vi "HDI Pat Match Full with Move TR.vi"(5 "controller in":refnum<k24>, 11 "error in":errorcluster) -> (4 "In Range?":bool, 8 "x rel move":dbl, 10 "y rel move":dbl, 14 "Horizontal vector":dbl[](array[numeric]), 15 "error out":errorcluster)   [LabVIEW 2011]
uses:
  C:/Users/Admin/Desktop/Gantry Code Transfer/source/Code Transfer/Aerotech.A3200.dll
  Aerotech.A3200.dll
  <vilib>/vision/driver/NI_Vision_Acquisition_Software.lvlib
panel:
  out "Angle Between Lines":dbl
  out "Diagnostic Log":string
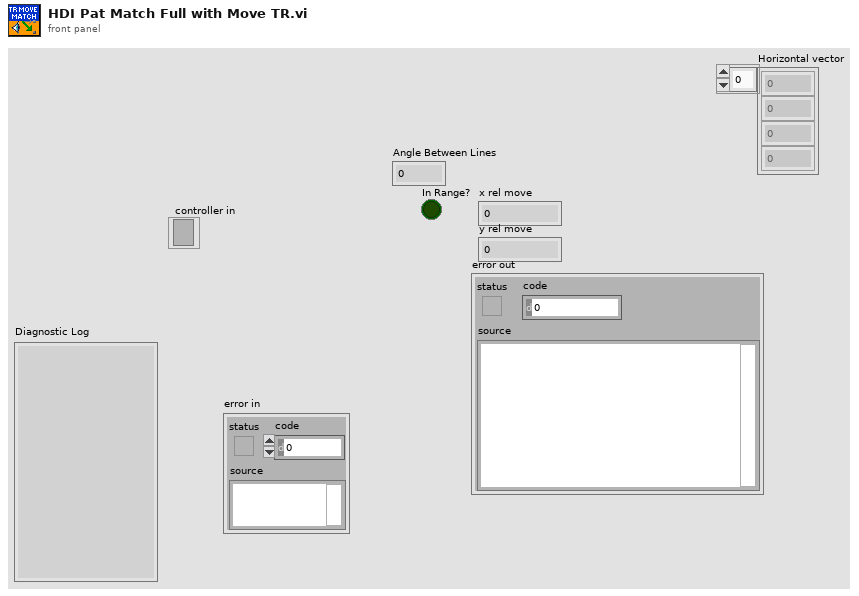
[diagram p1: front panel]
types:
  T1 = typedef "IMAQdx.ctl" = refnum<k21>
  T2 = typedef "IMAQ Image.ctl" = refnum<image>
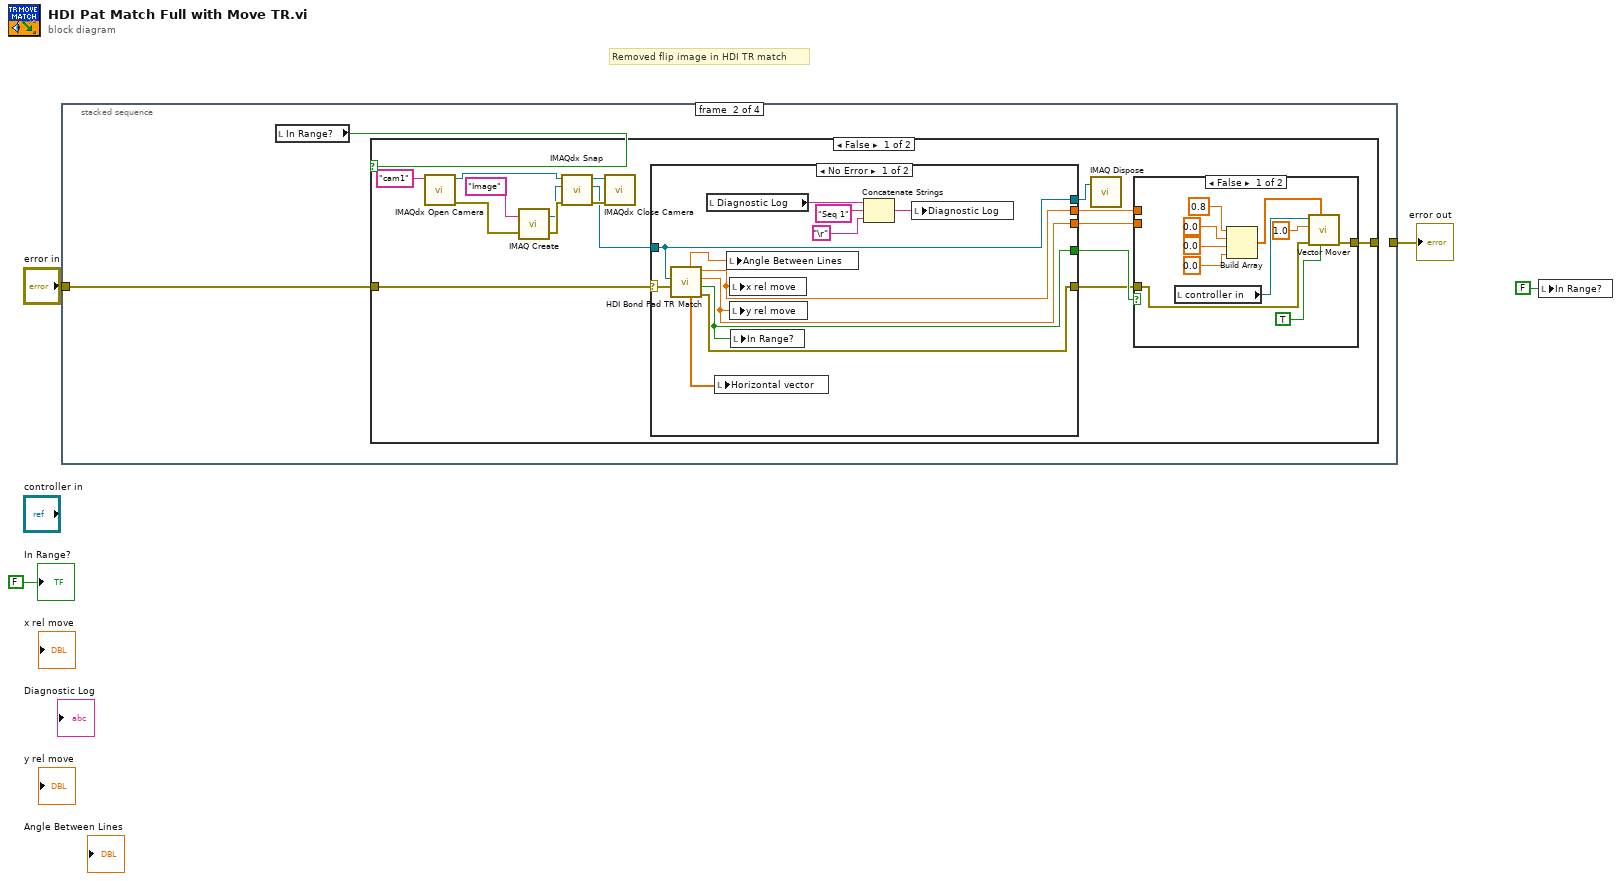
[diagram p0: block diagram]
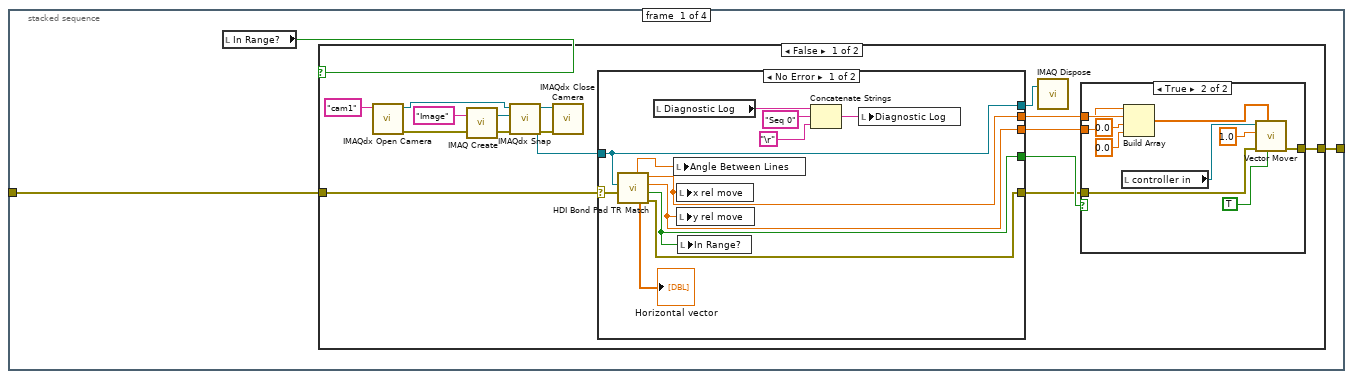
[diagram p2: hidden frame]
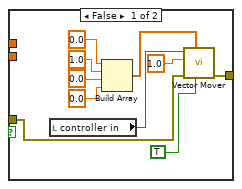
[diagram p3: hidden frame]
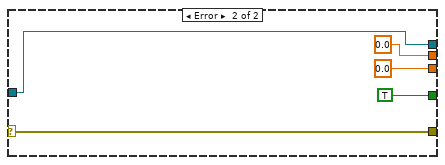
[diagram p4: hidden frame]
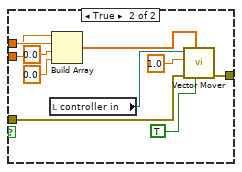
[diagram p6: hidden frame]
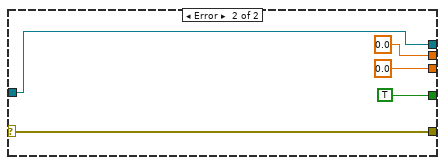
[diagram p7: hidden frame]
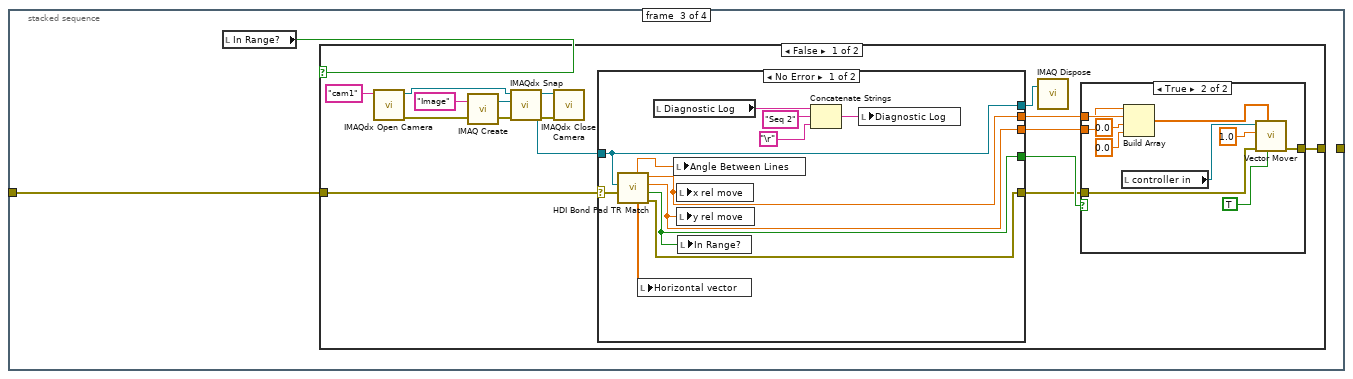
[diagram p9: hidden frame]
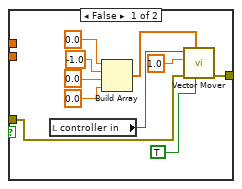
[diagram p10: hidden frame]
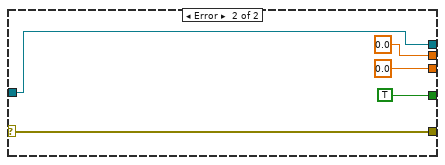
[diagram p11: hidden frame]
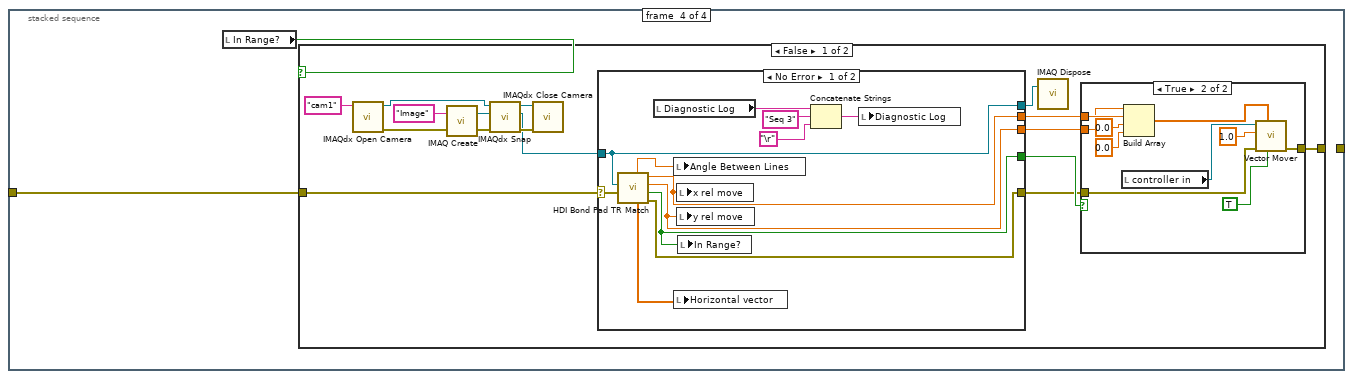
[diagram p13: hidden frame]
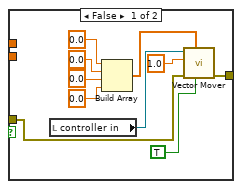
[diagram p14: hidden frame]
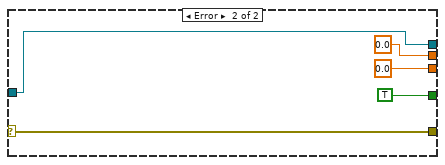
[diagram p15: hidden frame]
diagram:
  # "Removed flip image in HDI TR match"
  n1 = stacked-sequence {
    tunnel: "error in" -> [w7 w63 w119 w175]
    tunnel: [w6 _ _ _] -> w4
    frame #0 {
      n2 = local read "In Range?"() -> (w5:bool)
      n3 = case shown="False" w5 {
        tunnel: w7 -> [w23 w61]
        tunnel: [w20 w61] -> w6
        frame False {
          n4 = call <vilib>:"IMAQdx Open Camera.vi"("Session In"="cam1" ("Interface Name")) -> ("error out"=w14:errorcluster, "Session Out"=w9:T1)  [unwired: 9 in]
          n5 = call "IMAQ Create"("Image Name"="Image", "error in (no error)"=w14) -> ("New Image"=w11:T2, "error out"=w10:errorcluster)  [unwired: 3 in]
          n6 = call <vilib>:"IMAQdx Snap.vi"("error in"=w10, "Image In"=w11, "Session In"=w9) -> ("error out"=w12:errorcluster, "Image Out"=w8:T2, "Session Out"=w13:T1)  [unwired: 6 in]
          n7 = call <vilib>:"IMAQdx Close Camera.vi"("error in"=w12, "Session In"=w13) -> ()  [unwired: 9 in, 1 out]
          n8 = case shown="No Error" w23 {
            selector: w23 -> [w54 w60]
            tunnel: [w55 w60] -> w21
            tunnel: [w51 TRUE ("Matched?")] -> w22
            tunnel: [w53 0.0 ("x rel move")] -> w19
            tunnel: [w52 0.0 ("y rel move")] -> w18
            tunnel: w8 -> [w46 w56]
            tunnel: [w46 w56] -> w17
            frame No Error {
              n9 = call "HDI Bond Pad TR Match.vi"("error in (no error)"=w54, "Image Src"=w46) -> ("error out"=w55:errorcluster, "In Range?"=w51:bool, "y rel move"=w52:dbl, "x rel move"=w53:dbl, "Vertical vector"=→"Horizontal vector":dbl[], "Angle Between Lines"=w45:dbl)  [unwired: 4 in]
              n10 = local read "Diagnostic Log"() -> (w47:string)
              n11 = local write "Angle Between Lines"(w45) -> ()
              n12 = local write "x rel move"(w53) -> ()
              n13 = local write "y rel move"(w52) -> ()
              n14 = local write "In Range?"(w51) -> ()
              n15 = Concatenate Strings(w47, "Seq 0", "\r") -> (w50:string)
              n16 = local write "Diagnostic Log"(w50) -> ()
            }
            frame Error {
            }
          }
          n17 = call "IMAQ Dispose"("Image"=w17) -> ()  [unwired: 5 in, 1 out]
          n18 = case shown="True" w22 {
            tunnel: w21 -> [w31 w43]
            tunnel: [w26 w42] -> w20
            tunnel: w19 -> [_ w35]
            tunnel: w18 -> [_ w34]
            frame False {
              n19 = local read "controller in"() -> (w25:refnum<k24>)
              n20 = Build Array(0.0 ("element"), 1.0 ("element"), 0.0 ("element"), 0.0 ("element")) -> (w28:dbl[])
              n21 = call "Vector Mover.vi"("Absolute/Relative (F/T)"=TRUE, "Movement Vector"=w28, "error in (no error)"=w31, "Vector Speed"=1.0, "controller in"=w25) -> ("error out"=w26:errorcluster)  [unwired: 1 in, 3 out]
            }
            frame True {
              n22 = local read "controller in"() -> (w36:refnum<k24>)
              n23 = Build Array(w34, w35, 0.0 ("element"), 0.0 ("element")) -> (w37:dbl[])
              n24 = call "Vector Mover.vi"("Absolute/Relative (F/T)"=TRUE, "Movement Vector"=w37, "error in (no error)"=w43, "Vector Speed"=1.0, "controller in"=w36) -> ("error out"=w42:errorcluster)  [unwired: 1 in, 3 out]
            }
          }
        }
        frame True {
        }
      }
    }
    frame #1 {
      n25 = local read "In Range?"() -> (w62:bool)
      n26 = case shown="False" w62 {
        tunnel: w63 -> [w79 w117]
        tunnel: [w76 w117] -> _
        frame False {
          n27 = call <vilib>:"IMAQdx Open Camera.vi"("Session In"="cam1" ("Interface Name")) -> ("error out"=w67:errorcluster, "Session Out"=w72:T1)  [unwired: 9 in]
          n28 = call "IMAQ Create"("Image Name"="Image", "error in (no error)"=w67) -> ("New Image"=w70:T2, "error out"=w71:errorcluster)  [unwired: 3 in]
          n29 = call <vilib>:"IMAQdx Snap.vi"("error in"=w71, "Image In"=w70, "Session In"=w72) -> ("error out"=w69:errorcluster, "Image Out"=w64:T2, "Session Out"=w68:T1)  [unwired: 6 in]
          n30 = call <vilib>:"IMAQdx Close Camera.vi"("error in"=w69, "Session In"=w68) -> ()  [unwired: 9 in, 1 out]
          n31 = case shown="No Error" w79 {
            selector: w79 -> [w110 w116]
            tunnel: [w111 w116] -> w77
            tunnel: [w107 TRUE ("Matched?")] -> w78
            tunnel: [w109 0.0 ("x rel move")] -> w75
            tunnel: [w108 0.0 ("y rel move")] -> w74
            tunnel: w64 -> [w102 w112]
            tunnel: [w102 w112] -> w73
            frame No Error {
              n32 = call "HDI Bond Pad TR Match.vi"("error in (no error)"=w110, "Image Src"=w102) -> ("error out"=w111:errorcluster, "In Range?"=w107:bool, "y rel move"=w108:dbl, "x rel move"=w109:dbl, "Vertical vector"=w100:dbl[], "Angle Between Lines"=w101:dbl)  [unwired: 4 in]
              n33 = local read "Diagnostic Log"() -> (w103:string)
              n34 = local write "Horizontal vector"(w100) -> ()
              n35 = local write "Angle Between Lines"(w101) -> ()
              n36 = local write "x rel move"(w109) -> ()
              n37 = local write "y rel move"(w108) -> ()
              n38 = local write "In Range?"(w107) -> ()
              n39 = Concatenate Strings(w103, "Seq 1", "\r") -> (w106:string)
              n40 = local write "Diagnostic Log"(w106) -> ()
            }
            frame Error {
            }
          }
          n41 = call "IMAQ Dispose"("Image"=w73) -> ()  [unwired: 5 in, 1 out]
          n42 = case shown="False" w78 {
            tunnel: w77 -> [w87 w99]
            tunnel: [w81 w98] -> w76
            tunnel: w75 -> [_ w91]
            tunnel: w74 -> [_ w90]
            frame False {
              n43 = local read "controller in"() -> (w80:refnum<k24>)
              n44 = Build Array(0.8 ("element"), 0.0 ("element"), 0.0 ("element"), 0.0 ("element")) -> (w84:dbl[])
              n45 = call "Vector Mover.vi"("Absolute/Relative (F/T)"=TRUE, "Movement Vector"=w84, "error in (no error)"=w87, "Vector Speed"=1.0, "controller in"=w80) -> ("error out"=w81:errorcluster)  [unwired: 1 in, 3 out]
            }
            frame True {
              n46 = local read "controller in"() -> (w93:refnum<k24>)
              n47 = Build Array(w90, w91, 0.0 ("element"), 0.0 ("element")) -> (w92:dbl[])
              n48 = call "Vector Mover.vi"("Absolute/Relative (F/T)"=TRUE, "Movement Vector"=w92, "error in (no error)"=w99, "Vector Speed"=1.0, "controller in"=w93) -> ("error out"=w98:errorcluster)  [unwired: 1 in, 3 out]
            }
          }
        }
        frame True {
        }
      }
    }
    frame #2 {
      n49 = local read "In Range?"() -> (w118:bool)
      n50 = case shown="False" w118 {
        tunnel: w119 -> [w135 w173]
        tunnel: [w132 w173] -> _
        frame False {
          n51 = call <vilib>:"IMAQdx Open Camera.vi"("Session In"="cam1" ("Interface Name")) -> ("error out"=w126:errorcluster, "Session Out"=w121:T1)  [unwired: 9 in]
          n52 = call "IMAQ Create"("Image Name"="Image", "error in (no error)"=w126) -> ("New Image"=w123:T2, "error out"=w122:errorcluster)  [unwired: 3 in]
          n53 = call <vilib>:"IMAQdx Snap.vi"("error in"=w122, "Image In"=w123, "Session In"=w121) -> ("error out"=w124:errorcluster, "Image Out"=w120:T2, "Session Out"=w125:T1)  [unwired: 6 in]
          n54 = call <vilib>:"IMAQdx Close Camera.vi"("error in"=w124, "Session In"=w125) -> ()  [unwired: 9 in, 1 out]
          n55 = case shown="No Error" w135 {
            selector: w135 -> [w166 w172]
            tunnel: [w167 w172] -> w133
            tunnel: [w163 TRUE ("Matched?")] -> w134
            tunnel: [w165 0.0 ("x rel move")] -> w131
            tunnel: [w164 0.0 ("y rel move")] -> w130
            tunnel: w120 -> [w158 w168]
            tunnel: [w158 w168] -> w129
            frame No Error {
              n56 = call "HDI Bond Pad TR Match.vi"("error in (no error)"=w166, "Image Src"=w158) -> ("error out"=w167:errorcluster, "In Range?"=w163:bool, "y rel move"=w164:dbl, "x rel move"=w165:dbl, "Vertical vector"=w156:dbl[], "Angle Between Lines"=w157:dbl)  [unwired: 4 in]
              n57 = local write "Horizontal vector"(w156) -> ()
              n58 = local read "Diagnostic Log"() -> (w159:string)
              n59 = local write "Angle Between Lines"(w157) -> ()
              n60 = local write "x rel move"(w165) -> ()
              n61 = local write "y rel move"(w164) -> ()
              n62 = local write "In Range?"(w163) -> ()
              n63 = Concatenate Strings(w159, "Seq 2", "\r") -> (w162:string)
              n64 = local write "Diagnostic Log"(w162) -> ()
            }
            frame Error {
            }
          }
          n65 = call "IMAQ Dispose"("Image"=w129) -> ()  [unwired: 5 in, 1 out]
          n66 = case shown="True" w134 {
            tunnel: w133 -> [w143 w155]
            tunnel: [w137 w154] -> w132
            tunnel: w131 -> [_ w147]
            tunnel: w130 -> [_ w146]
            frame False {
              n67 = local read "controller in"() -> (w136:refnum<k24>)
              n68 = Build Array(0.0 ("element"), -1.0 ("element"), 0.0 ("element"), 0.0 ("element")) -> (w140:dbl[])
              n69 = call "Vector Mover.vi"("Absolute/Relative (F/T)"=TRUE, "Movement Vector"=w140, "error in (no error)"=w143, "Vector Speed"=1.0, "controller in"=w136) -> ("error out"=w137:errorcluster)  [unwired: 1 in, 3 out]
            }
            frame True {
              n70 = local read "controller in"() -> (w148:refnum<k24>)
              n71 = Build Array(w146, w147, 0.0 ("element"), 0.0 ("element")) -> (w149:dbl[])
              n72 = call "Vector Mover.vi"("Absolute/Relative (F/T)"=TRUE, "Movement Vector"=w149, "error in (no error)"=w155, "Vector Speed"=1.0, "controller in"=w148) -> ("error out"=w154:errorcluster)  [unwired: 1 in, 3 out]
            }
          }
        }
        frame True {
        }
      }
    }
    frame #3 {
      n73 = local read "In Range?"() -> (w174:bool)
      n74 = case shown="False" w174 {
        tunnel: w175 -> [w191 w229]
        tunnel: [w188 w229] -> _
        frame False {
          n75 = call <vilib>:"IMAQdx Open Camera.vi"("Session In"="cam1" ("Interface Name")) -> ("error out"=w182:errorcluster, "Session Out"=w177:T1)  [unwired: 9 in]
          n76 = call "IMAQ Create"("Image Name"="Image", "error in (no error)"=w182) -> ("New Image"=w179:T2, "error out"=w178:errorcluster)  [unwired: 3 in]
          n77 = call <vilib>:"IMAQdx Snap.vi"("error in"=w178, "Image In"=w179, "Session In"=w177) -> ("error out"=w180:errorcluster, "Image Out"=w176:T2, "Session Out"=w181:T1)  [unwired: 6 in]
          n78 = call <vilib>:"IMAQdx Close Camera.vi"("error in"=w180, "Session In"=w181) -> ()  [unwired: 9 in, 1 out]
          n79 = case shown="No Error" w191 {
            selector: w191 -> [w222 w228]
            tunnel: [w223 w228] -> w189
            tunnel: [w219 TRUE ("Matched?")] -> w190
            tunnel: [w221 0.0 ("x rel move")] -> w187
            tunnel: [w220 0.0 ("y rel move")] -> w186
            tunnel: w176 -> [w214 w224]
            tunnel: [w214 w224] -> w185
            frame No Error {
              n80 = call "HDI Bond Pad TR Match.vi"("error in (no error)"=w222, "Image Src"=w214) -> ("error out"=w223:errorcluster, "In Range?"=w219:bool, "y rel move"=w220:dbl, "x rel move"=w221:dbl, "Vertical vector"=w212:dbl[], "Angle Between Lines"=w213:dbl)  [unwired: 4 in]
              n81 = local read "Diagnostic Log"() -> (w215:string)
              n82 = local write "Angle Between Lines"(w213) -> ()
              n83 = local write "Horizontal vector"(w212) -> ()
              n84 = local write "x rel move"(w221) -> ()
              n85 = local write "y rel move"(w220) -> ()
              n86 = local write "In Range?"(w219) -> ()
              n87 = Concatenate Strings(w215, "Seq 3", "\r") -> (w218:string)
              n88 = local write "Diagnostic Log"(w218) -> ()
            }
            frame Error {
            }
          }
          n89 = call "IMAQ Dispose"("Image"=w185) -> ()  [unwired: 5 in, 1 out]
          n90 = case shown="True" w190 {
            tunnel: w189 -> [w199 w211]
            tunnel: [w193 w210] -> w188
            tunnel: w187 -> [_ w203]
            tunnel: w186 -> [_ w202]
            frame False {
              n91 = local read "controller in"() -> (w192:refnum<k24>)
              n92 = Build Array(0.0 ("element"), 0.0 ("element"), 0.0 ("element"), 0.0 ("element")) -> (w196:dbl[])
              n93 = call "Vector Mover.vi"("Absolute/Relative (F/T)"=TRUE, "Movement Vector"=w196, "error in (no error)"=w199, "Vector Speed"=1.0, "controller in"=w192) -> ("error out"=w193:errorcluster)  [unwired: 1 in, 3 out]
            }
            frame True {
              n94 = local read "controller in"() -> (w204:refnum<k24>)
              n95 = Build Array(w202, w203, 0.0 ("element"), 0.0 ("element")) -> (w205:dbl[])
              n96 = call "Vector Mover.vi"("Absolute/Relative (F/T)"=TRUE, "Movement Vector"=w205, "error in (no error)"=w211, "Vector Speed"=1.0, "controller in"=w204) -> ("error out"=w210:errorcluster)  [unwired: 1 in, 3 out]
            }
          }
        }
        frame True {
        }
      }
    }
  }
  "error out" <- w4
  n97 = local write "In Range?"(FALSE ("In Range?")) -> ()
  "In Range?" <- FALSE ("In Range?")
